vi "Run Test.vi"(8 "error in (no error)":errorcluster, 11 "Test Template in":refnum<class "Rocom Reset.lvclass">) -> (0 "error out":errorcluster, 1 "Fail Codes":string[](array[string]), 2 "Tests Passed":bool[](array[boolean]), 3 "Test Template out":refnum<class "Rocom Reset.lvclass">)   [LabVIEW 2015, in "Rocom Reset.lvclass"]
uses:
  Rocom Reset.lvclass
  Test Class/Test Class.lvclass
  Classes/Application/Class/Application.lvclass
  Rocom Tests/Rocom Tests.lvclass
  Classes/Manufacturing Test/Class/SC Manufacturing Test.lvclass
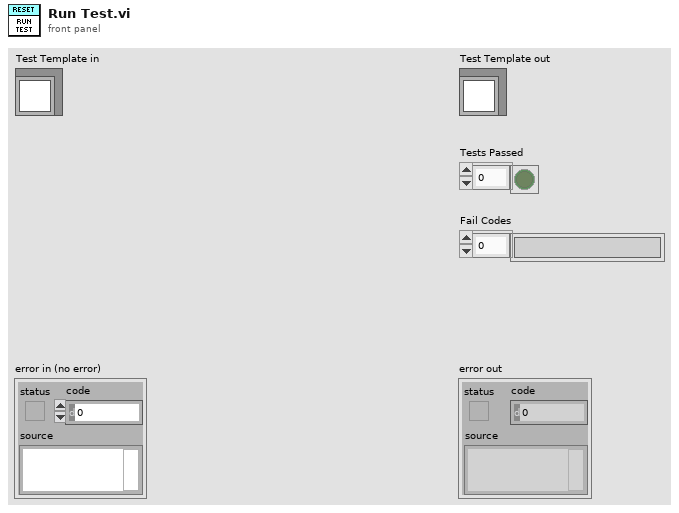
[diagram p1: front panel]
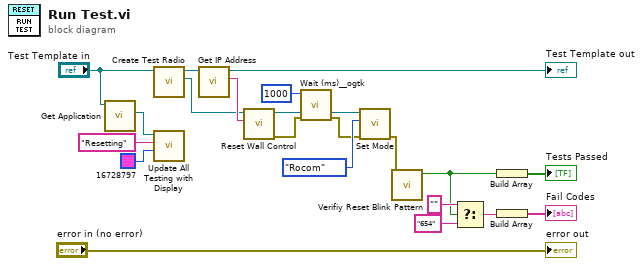
[diagram p0: block diagram]
diagram:
  n1 = call "Get Application.vi"("Test Class in"="Test Template in") -> ("Application.lvlib:Application.lvclass"=w21:refnum<class "Application.lvclass">)  [unwired: 9 in, 1 out]
  n2 = call "Create Test Radio.vi"("Rocom Tests in"="Test Template in") -> ("Test Radio"=w13:refnum<class "SC Manufacturing Test.lvclass">, "Rocom Tests out"=w15:refnum<class "Rocom Reset.lvclass">)  [unwired: 8 in, 1 out]
  n3 = call "Update All Testing with Display.vi"("BG Color"=u32 16728797, "Message ('')"="Resetting", "Application in"=w21) -> ()  [unwired: 7 in, 2 out]
  n4 = call "Get IP Address.vi"("Rocom Tests in"=w15) -> ("IP Address"=w14:string, "Rocom Tests out"=→"Test Template out":refnum<class "Rocom Reset.lvclass">)  [unwired: 8 in, 1 out]
  n5 = call "Reset Wall Control.vi"("IP Address"=w14, "Acrobat Template in"=w13) -> ("error out"=w3:errorcluster, "Acrobat Template out"=w16:refnum<class "SC Manufacturing Test.lvclass">)  [unwired: 8 in]
  n6 = call <userlib>:"Wait (ms)__ogtk.vi"("error in (no error)"=w3, "milliseconds to wait"=u32 1000) -> ("error out"=w2:errorcluster)  [unwired: 8 in, 1 out]
  n7 = call "Set Mode.vi"("error in (no error)"=w2, "Mode"=enum16{"Normal", "Test", "Rocom"}."Rocom", "Acrobat Template in"=w16) -> ("error out"=w4:errorcluster)  [unwired: 7 in, 1 out]
  n8 = call "Verifiy Reset Blink Pattern.vi"("Error in"=w4) -> ("Pass"=w5:bool)  [unwired: 9 in, 1 out]
  n9 = Select(t="", s=w5, f="654") -> (s? t:f=w10:string)
  n10 = Build Array(w5) -> (→"Tests Passed":bool[])
  n11 = Build Array(w10) -> (→"Fail Codes":string[])
  "error out" <- "error in (no error)"
